vi "Log Time.vi"(8 "error in (no error)":errorcluster, 10 "tdms file":refnum<k34>, 11 "Mag Lab Result in":refnum<class "Mag Lab Result.lvclass">) -> (0 "error out":errorcluster, 2 "tdms file out":refnum<k34>, 3 "Mag Lab Result out":refnum<class "Mag Lab Result.lvclass">)   [LabVIEW 2015, in "Mag Lab Result.lvclass"]
uses:
  Mag Lab Result.lvclass
  Mag Lab Result.lvclass/Mag Lab Result.ctl
  Read Group Name.vi
  Read Name.vi
  Read Result time.vi
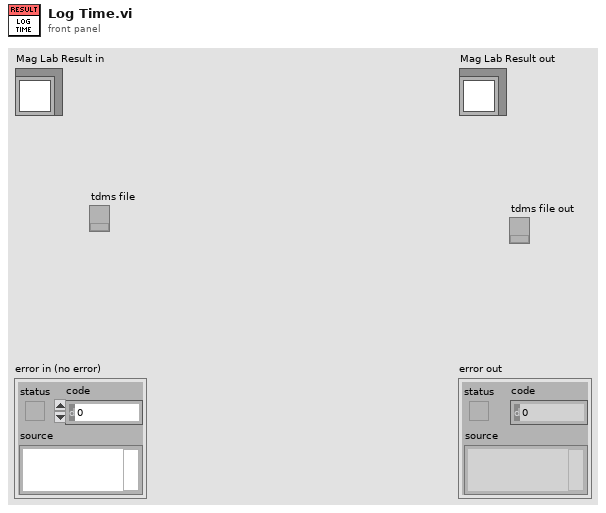
[diagram p1: front panel]
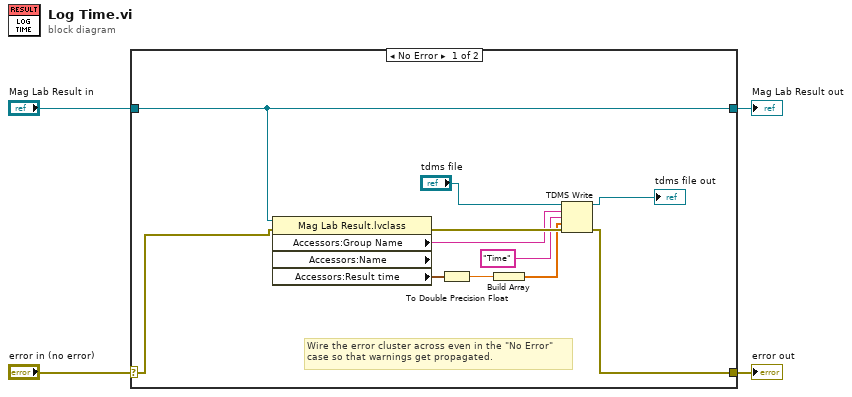
[diagram p0: block diagram]
diagram:
  n1 = case shown="No Error" "error in (no error)" {
    selector: "error in (no error)" -> [w6 w17]
    tunnel: [w7 w17] -> w3
    tunnel: [w10 w16] -> w1
    tunnel: "Mag Lab Result in" -> [w10 w16]
    frame No Error {
      # "Wire the error cluster across even in the \"No Error\"\ncase so that warnings get propagated."
      n2 = property class="Mag Lab Result.lvclass" props=["Accessors:Group Name", "Accessors:Name", "Accessors:Result time"](reference=w10, error in=w6) -> (error out=w15:errorcluster, "Accessors:Group Name"=w14:string, "Accessors:Result time"=w13:timestamp)  [unwired: 2 out]
      n3 = To Double Precision Float(number=w13) -> (double precision float=w11:dbl)
      n4 = Build Array(w11) -> (w12:dbl[])
      n5 = TDMS Write(0:"tdms file", 5:w14, 7:"Time", 9:w12, 11:w15) -> (4:→"tdms file out":refnum<k34>, 15:w7:errorcluster)  [unwired: 1 in, 2 out]
    }
    frame Error {
    }
  }
  "error out" <- w3
  "Mag Lab Result out" <- w1
